vi "Read ROI XY.vi"(8 "error in (no error)":errorcluster, 11 "TG Base Graph in":refnum<class "TG Base Graph.lvclass">) -> (0 "error out":errorcluster, 2 "ROI XY":T1, 3 "TG Base Graph out":refnum<class "TG Base Graph.lvclass">)   [LabVIEW 2023]
uses:
  TG Base Graph.lvclass
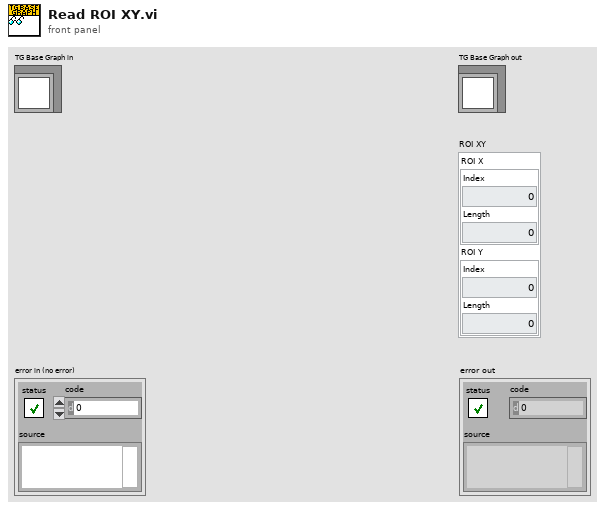
[diagram p1: front panel]
types:
  T1 = cluster{"ROI X":cluster{"Index":u32, "Length":u32}, "ROI Y":cluster{"Index":u32, "Length":u32}}
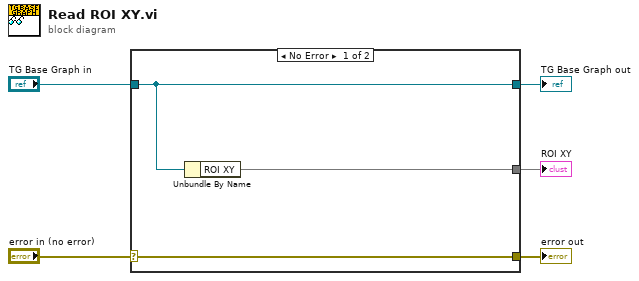
[diagram p0: block diagram]
diagram:
  n1 = case shown="No Error" "error in (no error)" {
    selector: "error in (no error)" -> [w8 w9]
    tunnel: [w8 w9] -> w4
    tunnel: [w7 w10] -> w2
    tunnel: "TG Base Graph in" -> [w7 w10]
    tunnel: [w6 _] -> w1
    frame No Error {
      n2 = Unbundle By Name(w7) -> ("ROI XY"=w6)
    }
    frame Error {
    }
  }
  "error out" <- w4
  "TG Base Graph out" <- w2
  "ROI XY" <- w1
